vi "init.vi"(8 "error in":errorcluster, 10 "TBM module configuration in":refnum<class "TBM module configuration.lvclass">, 11 "Daqmx Module runtime in":refnum<class "DAQmx Module Runtime.lvclass">) -> (0 "error out":errorcluster, 1 "data allocations":T1, 2 "execution settings":T4, 3 "Daqmx Module runtime out":refnum<class "DAQmx Module Runtime.lvclass">)   [LabVIEW 2015, in "DAQmx Module Runtime.lvclass"]
doc: "Provides an interface for initializing a module at runtime. While this interface performs no operations, a child should provide an override which may open any necessary references or sessions, allocate necessary memory, and perform any final configuration validataion before providing the full configuration <b>execution data</b> to the calling process."
uses:
  DAQmx Module Runtime.lvclass
  <vilib>/NI/Tag Bus Module Framework/module configuration/TBM module configuration.lvclass
  <vilib>/NI/Tag Bus Module Framework/runtime/execution settings.ctl
  <vilib>/NI/Tag Bus Module Framework/channel/data tables.ctl
  <vilib>/NI/Tag Bus/dictionary/data dictionary.lvclass
  <vilib>/NI/Tag Bus/dictionary table pair.ctl
  <vilib>/NI/Tag Bus/table/data table.ctl
  configuration/Daqmx Module configuration.lvclass
  Channel Indeces.ctl
  configuration/Daqmx Module configuration.lvclass/Daqmx Module configuration.ctl
  <vilib>/NI/Tag Bus/tag/tag descriptor.lvclass/tag descriptor.ctl
  DAQmx Module Runtime.lvclass/DAQmx Module Runtime.ctl
  configuration/Read Data Rate.vi
  <vilib>/NI/Tag Bus/tag/read tag name.vi
  <vilib>/NI/Tag Bus/tag/read data type.vi
  <vilib>/NI/Tag Bus/dictionary/locate tag.vi
  <vilib>/DAQmx/create/channels.llb/DAQmx Create Channel (AI-Voltage-Basic).vi
  <vilib>/DAQmx/create/channels.llb/DAQmx Create Channel (AI-Strain-Strain Gage).vi
  <vilib>/DAQmx/create/channels.llb/DAQmx Create Channel (AI-Temperature-Thermocouple).vi
  <vilib>/DAQmx/create/channels.llb/DAQmx Create Channel (AI-Current-Basic).vi
  <vilib>/DAQmx/create/channels.llb/DAQmx Create Channel (AI-Temperature-RTD).vi
  <vilib>/DAQmx/create/channels.llb/DAQmx Create Channel (AO-Current-Basic).vi
  <vilib>/DAQmx/create/channels.llb/DAQmx Create Channel (AO-Voltage-Basic).vi
  <vilib>/DAQmx/create/channels.llb/DAQmx Create Channel (DO-Digital Output).vi
  <vilib>/DAQmx/create/channels.llb/DAQmx Create Channel (CO-Pulse Generation-Frequency).vi
  <vilib>/DAQmx/create/channels.llb/DAQmx Create Channel (DI-Digital Input).vi
  <vilib>/NI/Tag Bus Module Framework/channel/TBM channel.lvclass
  <vilib>/NI/Tag Bus Module Framework/runtime/TBM module execution interface.lvclass
  <resource>/objmgr/daqmx.rc
  <vilib>/NI/Tag Bus/tag bus.lvlib
  <vilib>/NI/Tag Bus/table/data table.lvlib
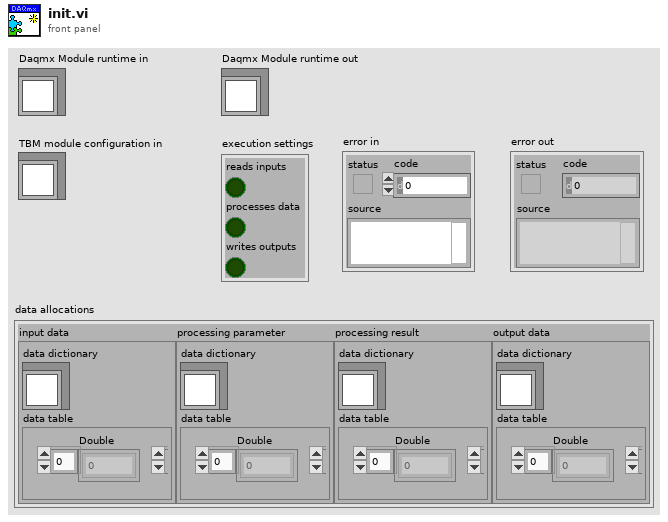
[diagram p1: front panel]
types:
  T1 = typedef "TBM channel.lvclass/data tables.ctl" = cluster{"input data":T2, "processing parameter":T2, "processing result":T2, "output data":T2}
  T2 = typedef "tag bus.lvlib/dictionary table pair.ctl" = cluster{"data dictionary":refnum<class "data dictionary.lvclass">, "data table":T3}
  T3 = typedef "tag bus.lvlib/data table.lvlib/data table.ctl" = cluster{"Double":dbl[], "Single":sgl[], "I64":i64[], "I32":i32[], "I16":i16[], "I8":i8[], "U64":u64[], "U32":u32[], "U16":u16[], "U8":u8[], "Boolean":bool[], "String":string[], "Array of Double":cluster{"DBL Array":dbl[]}[], "Array of Single":cluster{"SGL Array":sgl[]}[], "Array of I64":cluster{"I64 Array":i64[]}[], "Array of I32":cluster{"I32 Array":i32[]}[], "Array of I16":cluster{"I16 Array":i16[]}[], "Array of I8":cluster{"I8 Array":i8[]}[], "Array of U64":cluster{"U64 Array":u64[]}[], "Array of U32":cluster{"U32 Array":u32[]}[], "Array of U16":cluster{"U16 Array":u16[]}[], "Array of U8":cluster{"U8 Array":u8[]}[], "Array of Boolean":cluster{"Boolean Array":bool[]}[], "Array of String":cluster{"String Array":string[]}[]}
  T4 = typedef "TBM module execution interface.lvclass/execution settings.ctl" = cluster{"reads inputs":bool, "processes data":bool, "writes outputs":bool}
  T5 = typedef "DAQmx Module Runtime.lvclass/Channel Indeces.ctl" = cluster{"AI Index":i32[], "AO Index":i32[], "DI Index":i32[], "DO Index":i32[], "PWM Freq Index":i32[], "PWM DC Index":i32[]}
  T6 = typedef "DAQmx Module Configuration.lvclass/Line.ctl" = cluster{"Channel Array":refnum<class "TBM channel.lvclass">[], "Physical Channel":string, "Measurement Type":T7, "Parameters":T8}
  T7 = typedef "DAQmx Module Configuration.lvclass/Measurement Type.ctl" = enum16{"Digital Input", "Digital Output", "Voltage Input", "Voltage Output", "Current Input", "Current Output", "RTD", "Thermocouple", "Strain", "PWM"}
  T8 = typedef "DAQmx Module Configuration.lvclass/Parameters.ctl" = cluster{"Digital Config":cluster{"Invert Lines?":bool}, "Voltage Config":cluster{"Maximum Value (V)":dbl, "Minimum Value (V)":dbl, "in terminal configuration (V)":i32, "out terminal configuration (V)":i32}, "Current Config":cluster{"Maximum Value (A)":dbl, "Minimum Value (A)":dbl, "shunt resistor location":i32, "input terminal configuration (C)":i32, "external shunt resistor value":dbl}, "RTD Config":cluster{"Maximum Value (°C)":dbl, "Minimum Value (°C)":dbl, "resistance configuration":i32, "r0":dbl, "current excitation value":dbl, "rtd type":i32, "current excitation source":i32}, "Thermocouple Config":cluster{"Minimum Value (C)":dbl, "Maximum Value (C)":dbl, "thermocouple type":i32, "cjc source":i32, "cjc value":dbl}, "Strain Config":cluster{"Maximum Value":dbl, "Minimum Value":dbl, "bridge information":cluster{"strain configuration":i32, "lead wire resistance":dbl, "initial bridge voltage":dbl, "voltage excitation source":i32, "voltage excitation value":dbl}, "strain gage information":cluster{"gage factor":dbl, "nominal gage resistance":dbl, "poisson ratio":dbl}}, "PWM Config":cluster{"Idle State":bool}}
  T9 = typedef "DAQmx Module Runtime.lvclass/DAQ Tasks.ctl" = cluster{"AI Task":refnum<k21>, "AO Task":refnum<k21>, "DI Task":refnum<k21>, "DO Task":refnum<k21>, "PWM Task":refnum<k21>}
  T10 = cluster{"strain configuration":i32, "lead wire resistance":dbl, "initial bridge voltage":dbl, "voltage excitation source":i32, "voltage excitation value":dbl}
  T11 = cluster{"gage factor":dbl, "nominal gage resistance":dbl, "poisson ratio":dbl}
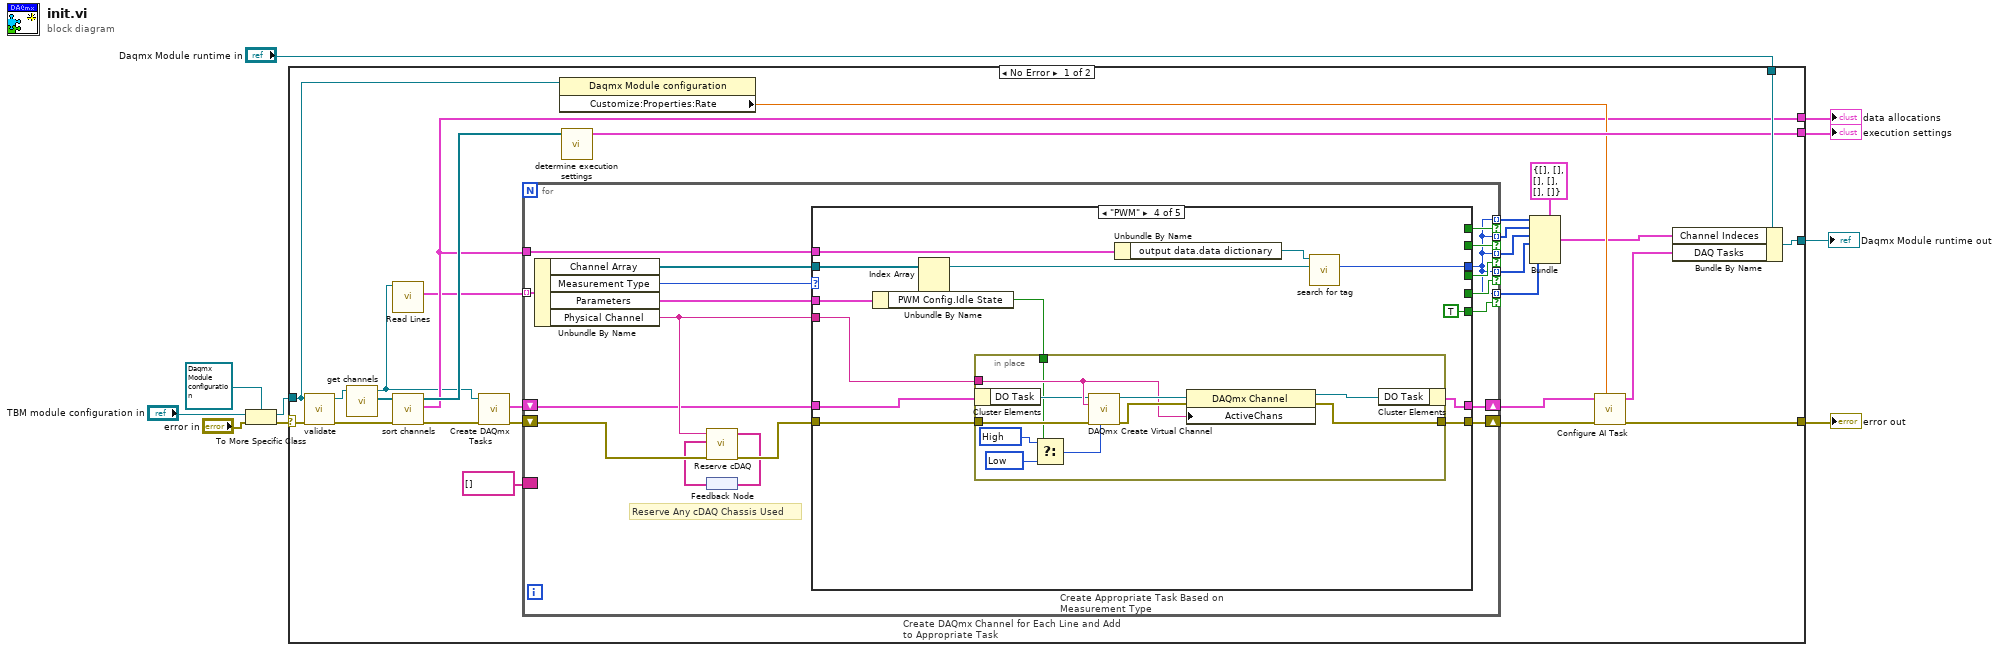
[diagram p0: block diagram]
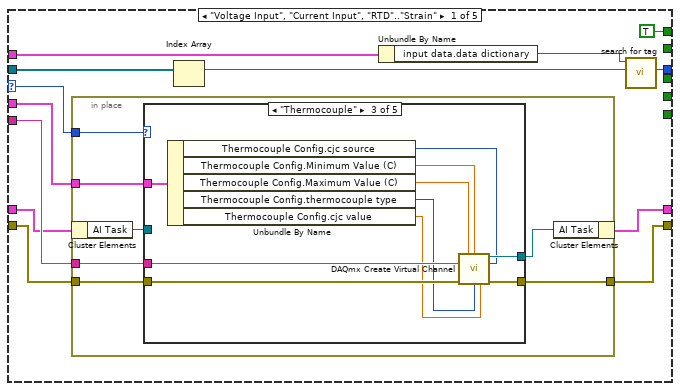
[diagram p2: hidden frame]
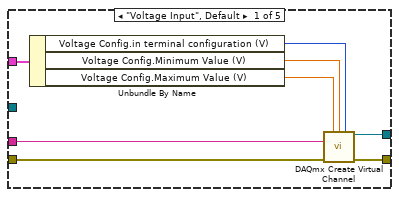
[diagram p3: hidden frame]
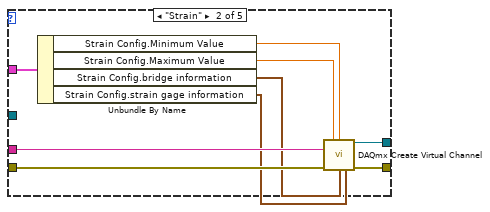
[diagram p4: hidden frame]
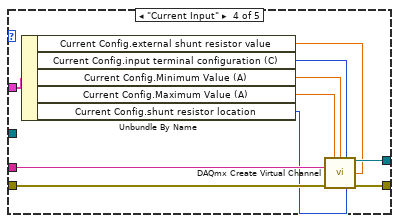
[diagram p5: hidden frame]
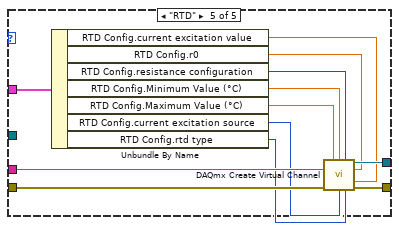
[diagram p6: hidden frame]
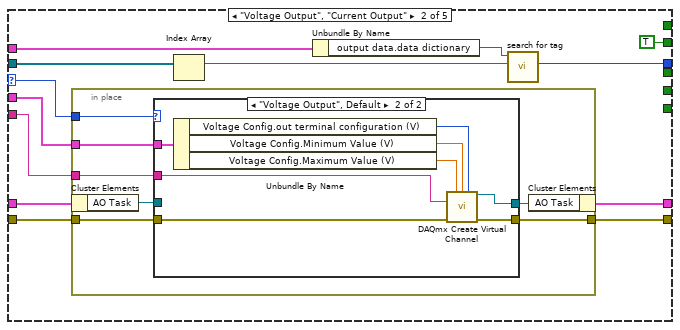
[diagram p7: hidden frame]
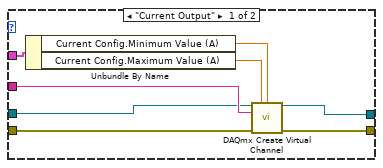
[diagram p8: hidden frame]
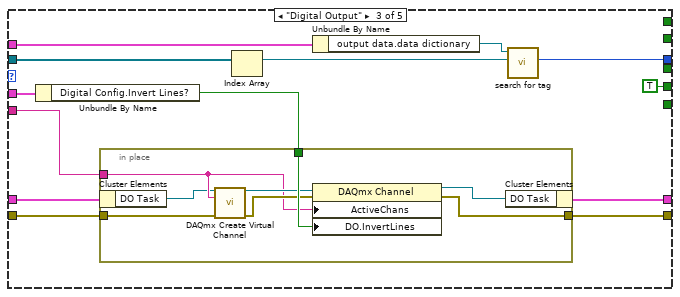
[diagram p9: hidden frame]
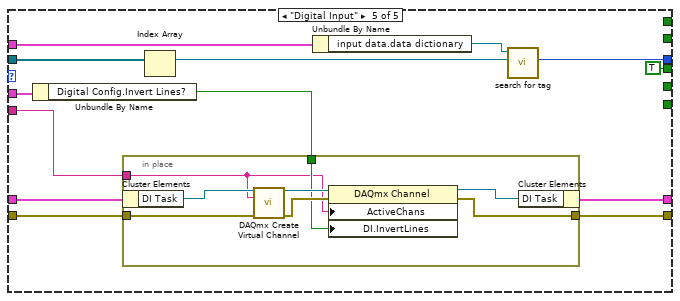
[diagram p10: hidden frame]
diagram:
  n1 = To More Specific Class(target class=refnum<class "Daqmx Module configuration.lvclass"> refnum ("Synchronous module configuration"), reference="TBM module configuration in", error in="error in") -> (specific class reference=w9:refnum<class "Daqmx Module configuration.lvclass">, error out=w10:errorcluster)
  n2 = case shown="No Error" w10 {
    selector: w10 -> [w34 w230]
    tunnel: w9 -> [w30 _]
    tunnel: "Daqmx Module runtime in" -> [w38 w229]
    tunnel: [w31 w229] -> w6
    tunnel: [w19 w230] -> w5
    tunnel: [w14 _] -> w3
    tunnel: [w37 _] -> w4
    frame No Error {
      n3 = call-dynamic "validate.vi"("error in"=w34, "Daqmx Module configuration in"=w30) -> ("error out"=w35:errorcluster, "Daqmx Module configuration out"=w33:refnum<class "Daqmx Module configuration.lvclass">)  [unwired: 8 in]
      n4 = call-dynamic "get channels.vi"("Daqmx Module configuration in"=w33) -> ("channels"=w32:refnum<class "TBM channel.lvclass">[], "Daqmx Module configuration out"=w13:refnum<class "Daqmx Module configuration.lvclass">)  [unwired: 9 in]
      n5 = call "Read Lines.vi"("Daqmx Module configuration in"=w13) -> ("Lines"=w12:T6[])  [unwired: 8 in, 2 out]
      n6 = call <vilib>:"sort channels.vi"("error in"=w35, "channels in"=w32) -> ("error out"=w29:errorcluster, "data allocations"=w14:T1, "channels out"=w36:refnum<class "TBM channel.lvclass">[])  [unwired: 7 in]
      n7 = call "Create DAQmx Tasks.vi"("Error In"=w29, "Daqmx Module configuration"=w13) -> ("Error Out"=w28:errorcluster, "DAQ Tasks"=w27:T9)  [unwired: 8 in]
      n8 = for "Create DAQmx Channel for Each Line and Add to Appropriate Task" {
        shift-right: [w45] -> w20
        shift-left: w28 -> [w47]
        tunnel: w12 -> [w57] mode=indexing
        tunnel: w14 -> [w55]
        tunnel: [w40] -> w21 mode=indexing if=w54
        tunnel: [w40] -> w22 mode=indexing if=w52
        tunnel: [w40] -> w24 mode=indexing if=w50
        tunnel: [w40] -> w23 mode=indexing if=w51
        shift-right: [w41] -> w18
        shift-left: w27 -> [w44]
        border: string[] [] -> [_]
        tunnel: [w40] -> w11 mode=indexing if=w39
        # "Reserve Any cDAQ Chassis Used"
        n9 = Unbundle By Name(w57) -> ("Channel Array"=w49:refnum<class "TBM channel.lvclass">[], "Measurement Type"=w56:T7, "Parameters"=w53:T8, "Physical Channel"=w48:string)
        n10 = feedback #1() -> (w42:string[])
        n11 = call "Reserve cDAQ.vi"("error in (no error)"=w47, "Array in"=w42, "Physical Channel"=w48) -> ("error out"=w46:errorcluster, "Array out"=w43:string[])  [unwired: 7 in]
        n12 = feedback-in #1(w43) -> ()
        n13 = case "Create Appropriate Task Based on Measurement Type" shown="\"PWM\"" w56 {
          selector: w56 -> [w64 w132 _ _ _]
          tunnel: w46 -> [w70 w139 w175 w196 w220]
          tunnel: [w62 w138 w168 w191 w214] -> w45
          tunnel: w55 -> [w69 w137 w174 w195 w219]
          tunnel: [_ _ TRUE _ _] -> w54
          tunnel: w49 -> [w68 w136 w173 w194 w218]
          tunnel: [w67 w135 w172 w193 w217] -> w40
          tunnel: w53 -> [w63 w131 w170 w187 w215]
          tunnel: [_ _ _ _ TRUE] -> w52
          tunnel: [_ TRUE _ _ _] -> w51
          tunnel: [TRUE _ _ _ _] -> w50
          tunnel: w48 -> [w65 w133 w167 w190 w213]
          tunnel: w44 -> [w61 w130 w166 w189 w211]
          tunnel: [w60 w129 w165 w188 w210] -> w41
          tunnel: [_ _ _ TRUE _] -> w39
          frame "Voltage Input", "Current Input", "RTD".."Strain" {
            n14 = in-place {
              in-place-border: w70 -> [w77]
              in-place-border: w65 -> [w76]
              in-place-border: w64 -> [w75]
              in-place-border: w63 -> [w74]
              in-place-border: [w73] -> w62
              n15 = in-place-cluster #2(w61) -> ("AI Task"=w72:refnum<k21>)
              n16 = case shown="\"Thermocouple\"" w75 {
                tunnel: w77 -> [w85 w94 w104 w114 w126]
                tunnel: [w84 w93 w103 w113 w125] -> w73
                tunnel: [w83 w92 w102 w112 w124] -> w71
                tunnel: w76 -> [w82 w91 w101 w111 w123]
                tunnel: w74 -> [w80 w89 w99 w109 w122]
                tunnel: w72 -> [_ _ _ _ _]
                frame "Voltage Input", Default {
                  n17 = Unbundle By Name(w80) -> ("Voltage Config.in terminal configuration (V)"=w78:i32, "Voltage Config.Minimum Value (V)"=w79:dbl, "Voltage Config.Maximum Value (V)"=w81:dbl)
                  n18 = call-poly <vilib>:"DAQmx Create Virtual Channel.vi"("maximum value"=w81, "minimum value"=w79, "input terminal configuration"=w78, "physical channels"=w82, "error in"=w85) -> ("task out"=w83:refnum<k21>, "error out"=w84:errorcluster)  [unwired: 9 in]
                }
                frame "Strain" {
                  n19 = Unbundle By Name(w89) -> ("Strain Config.Minimum Value"=w88:dbl, "Strain Config.Maximum Value"=w90:dbl, "Strain Config.bridge information"=w87:T10, "Strain Config.strain gage information"=w86:T11)
                  n20 = call-poly <vilib>:"DAQmx Create Virtual Channel.vi"("maximum value"=w90, "minimum value"=w88, "physical channels"=w91, "error in"=w94, "bridge information"=w87, "strain gage information"=w86) -> ("task out"=w92:refnum<k21>, "error out"=w93:errorcluster)  [unwired: 8 in]
                }
                frame "Thermocouple" {
                  n21 = Unbundle By Name(w99) -> ("Thermocouple Config.cjc source"=w95:i32, "Thermocouple Config.Minimum Value (C)"=w98:dbl, "Thermocouple Config.Maximum Value (C)"=w100:dbl, "Thermocouple Config.thermocouple type"=w97:i32, "Thermocouple Config.cjc value"=w96:dbl)
                  n22 = call-poly <vilib>:"DAQmx Create Virtual Channel.vi"("maximum value"=w100, "minimum value"=w98, "physical channels"=w101, "cjc source"=w95, "error in"=w104, "thermocouple type"=w97, "cjc value"=w96) -> ("task out"=w102:refnum<k21>, "error out"=w103:errorcluster)  [unwired: 7 in]
                }
                frame "Current Input" {
                  n23 = Unbundle By Name(w109) -> ("Current Config.external shunt resistor value"=w106:dbl, "Current Config.input terminal configuration (C)"=w107:i32, "Current Config.Minimum Value (A)"=w108:dbl, "Current Config.Maximum Value (A)"=w110:dbl, "Current Config.shunt resistor location"=w105:i32)
                  n24 = call-poly <vilib>:"DAQmx Create Virtual Channel.vi"("maximum value"=w110, "minimum value"=w108, "input terminal configuration"=w107, "physical channels"=w111, "external shunt resistor value"=w106, "error in"=w114, "shunt resistor location"=w105) -> ("task out"=w112:refnum<k21>, "error out"=w113:errorcluster)  [unwired: 7 in]
                }
                frame "RTD" {
                  n25 = Unbundle By Name(w122) -> ("RTD Config.current excitation value"=w117:dbl, "RTD Config.r0"=w116:dbl, "RTD Config.resistance configuration"=w119:i32, "RTD Config.Minimum Value (°C)"=w120:dbl, "RTD Config.Maximum Value (°C)"=w121:dbl, "RTD Config.current excitation source"=w118:i32, "RTD Config.rtd type"=w115:i32)
                  n26 = call-poly <vilib>:"DAQmx Create Virtual Channel.vi"("maximum value"=w121, "minimum value"=w120, "resistance configuration"=w119, "physical channels"=w123, "r0"=w116, "current excitation value"=w117, "error in"=w126, "current excitation source"=w118, "rtd type"=w115) -> ("task out"=w124:refnum<k21>, "error out"=w125:errorcluster)  [unwired: 5 in]
                }
              }
              n27 = in-place-cluster #2("AI Task"=w71) -> (w60:T9)
            }
            n28 = Index Array(array=w68) -> (element=w58:refnum<class "TBM channel.lvclass">)  [unwired: 1 in]
            n29 = Unbundle By Name(w69) -> ("input data.data dictionary"=w66:refnum<class "data dictionary.lvclass">)
            n30 = call <vilib>:"search for tag.vi"("system tag"=w58, "data dictionary in"=w66) -> ("index"=w67:i32)  [unwired: 7 in, 2 out]
          }
          frame "Voltage Output", "Current Output" {
            n31 = in-place {
              in-place-border: w139 -> [w146]
              in-place-border: [w145] -> w138
              in-place-border: w133 -> [w144]
              in-place-border: w132 -> [w143]
              in-place-border: w131 -> [w142]
              n32 = in-place-cluster #3(w130) -> ("AO Task"=w140:refnum<k21>)
              n33 = case shown="\"Voltage Output\", Default" w143 {
                tunnel: w146 -> [w154 w162]
                tunnel: [w153 w161] -> w141
                tunnel: [w152 w160] -> w145
                tunnel: w144 -> [w151 w159]
                tunnel: w142 -> [w150 w158]
                tunnel: w140 -> [w147 _]
                frame "Current Output" {
                  n34 = Unbundle By Name(w150) -> ("Current Config.Minimum Value (A)"=w148:dbl, "Current Config.Maximum Value (A)"=w149:dbl)
                  n35 = call-poly <vilib>:"DAQmx Create Virtual Channel.vi"("task in"=w147, "maximum value"=w149, "minimum value"=w148, "physical channels"=w151, "error in"=w154) -> ("task out"=w153:refnum<k21>, "error out"=w152:errorcluster)  [unwired: 9 in]
                }
                frame "Voltage Output", Default {
                  n36 = Unbundle By Name(w158) -> ("Voltage Config.out terminal configuration (V)"=w155:i32, "Voltage Config.Minimum Value (V)"=w156:dbl, "Voltage Config.Maximum Value (V)"=w157:dbl)
                  n37 = call-poly <vilib>:"DAQmx Create Virtual Channel.vi"("maximum value"=w157, "minimum value"=w156, "output terminal configuration"=w155, "physical channels"=w159, "error in"=w162) -> ("task out"=w161:refnum<k21>, "error out"=w160:errorcluster)  [unwired: 9 in]
                }
              }
              n38 = in-place-cluster #3("AO Task"=w141) -> (w129:T9)
            }
            n39 = Index Array(array=w136) -> (element=w127:refnum<class "TBM channel.lvclass">)  [unwired: 1 in]
            n40 = Unbundle By Name(w137) -> ("output data.data dictionary"=w134:refnum<class "data dictionary.lvclass">)
            n41 = call <vilib>:"search for tag.vi"("system tag"=w127, "data dictionary in"=w134) -> ("index"=w135:i32)  [unwired: 7 in, 2 out]
          }
          frame "Digital Output" {
            n42 = Unbundle By Name(w170) -> ("Digital Config.Invert Lines?"=w169:bool)
            n43 = in-place {
              in-place-border: w175 -> [w183]
              in-place-border: w169 -> [w182]
              in-place-border: [w179] -> w168
              in-place-border: w167 -> [w178]
              n44 = in-place-cluster #4(w166) -> ("DO Task"=w177:refnum<k21>)
              n45 = call-poly <vilib>:"DAQmx Create Virtual Channel.vi"("task in"=w177, "lines"=w178, "error in"=w183) -> ("task out"=w180:refnum<k21>, "error out"=w181:errorcluster)  [unwired: 11 in]
              n46 = property class="DAQmx Channel"(reference=w180, error in=w181, "ActiveChans"=w178, "DO.InvertLines"=w182) -> (reference out=w176:refnum<k21>, error out=w179:errorcluster)
              n47 = in-place-cluster #4("DO Task"=w176) -> (w165:T9)
            }
            n48 = Index Array(array=w173) -> (element=w163:refnum<class "TBM channel.lvclass">)  [unwired: 1 in]
            n49 = Unbundle By Name(w174) -> ("output data.data dictionary"=w171:refnum<class "data dictionary.lvclass">)
            n50 = call <vilib>:"search for tag.vi"("system tag"=w163, "data dictionary in"=w171) -> ("index"=w172:i32)  [unwired: 7 in, 2 out]
          }
          frame "PWM" {
            n51 = Unbundle By Name(w187) -> ("PWM Config.Idle State"=w186:bool)
            n52 = Index Array(array=w194) -> (element #1=w184:refnum<class "TBM channel.lvclass">)  [unwired: 2 in, 1 out]
            n53 = in-place {
              in-place-border: w196 -> [w207]
              in-place-border: [w204] -> w191
              in-place-border: w190 -> [w203]
              in-place-border: w186 -> [w198]
              w197 = 10214 items=["High"=10192, "Low"=10214] ("idle state")
              w200 = 10192 items=["High"=10192, "Low"=10214] ("idle state")
              n54 = in-place-cluster #5(w189) -> ("DO Task"=w202:refnum<k21>)
              n55 = Select(t=w200, s=w198, f=w197) -> (s? t:f=w199:i32)
              n56 = call-poly <vilib>:"DAQmx Create Virtual Channel.vi"("task in"=w202, "counter"=w203, "error in"=w207, "idle state"=w199) -> ("task out"=w205:refnum<k21>, "error out"=w206:errorcluster)  [unwired: 10 in]
              n57 = property class="DAQmx Channel"(reference=w205, error in=w206, "ActiveChans"=w203) -> (reference out=w201:refnum<k21>, error out=w204:errorcluster)
              n58 = in-place-cluster #5("DO Task"=w201) -> (w188:T9)
            }
            n59 = Unbundle By Name(w195) -> ("output data.data dictionary"=w192:refnum<class "data dictionary.lvclass">)
            n60 = call <vilib>:"search for tag.vi"("system tag"=w184, "data dictionary in"=w192) -> ("index"=w193:i32)  [unwired: 7 in, 2 out]
          }
          frame "Digital Input" {
            n61 = Unbundle By Name(w215) -> ("Digital Config.Invert Lines?"=w212:bool)
            n62 = in-place {
              in-place-border: w220 -> [w228]
              in-place-border: [w225] -> w214
              in-place-border: w213 -> [w221]
              in-place-border: w212 -> [w224]
              n63 = in-place-cluster #6(w211) -> ("DI Task"=w223:refnum<k21>)
              n64 = call-poly <vilib>:"DAQmx Create Virtual Channel.vi"("task in"=w223, "lines"=w221, "error in"=w228) -> ("task out"=w227:refnum<k21>, "error out"=w226:errorcluster)  [unwired: 11 in]
              n65 = property class="DAQmx Channel"(reference=w227, error in=w226, "ActiveChans"=w221, "DI.InvertLines"=w224) -> (reference out=w222:refnum<k21>, error out=w225:errorcluster)
              n66 = in-place-cluster #6("DI Task"=w222) -> (w210:T9)
            }
            n67 = Index Array(array=w218) -> (element=w208:refnum<class "TBM channel.lvclass">)  [unwired: 1 in]
            n68 = Unbundle By Name(w219) -> ("input data.data dictionary"=w216:refnum<class "data dictionary.lvclass">)
            n69 = call <vilib>:"search for tag.vi"("system tag"=w208, "data dictionary in"=w216) -> ("index"=w217:i32)  [unwired: 7 in, 2 out]
          }
        }
      }
      n70 = property class="Daqmx Module configuration"(reference=w30) -> ("Customize:Properties:Rate"=w17:dbl)  [unwired: 1 in, 2 out]
      n71 = call <vilib>:"determine execution settings.vi"("channels"=w36) -> ("execution settings"=w37:T4)  [unwired: 10 in]
      n72 = Bundle(cluster=T5 {"AI Index"=[], "AO Index"=[], "DI Index"=[], "DO Index"=[], "PWM Freq Index"=[], "PWM DC Index"=[]} ("Channel Indeces"), "AI Index"=w24, "AO Index"=w23, "DI Index"=w22, "DO Index"=w21, "PWM Freq Index"=w11) -> (w16:T5)  [unwired: 1 in]
      n73 = call "Configure AI Task.vi"("Sampling Rate"=w17, "error in (no error)"=w20, "DAQ Tasks in"=w18) -> ("error out"=w19:errorcluster, "DAQ Tasks out"=w15:T9)  [unwired: 7 in]
      n74 = Bundle By Name(cluster=w38, "Channel Indeces"=w16, "DAQ Tasks"=w15) -> (w31:refnum<class "DAQmx Module Runtime.lvclass">)
    }
    frame Error {
    }
  }
  "error out" <- w5
  "Daqmx Module runtime out" <- w6
  "execution settings" <- w4
  "data allocations" <- w3
